vi "example_01_binary_tree.vi"(8 "error in (no error)":errorcluster) -> (0 "error out":errorcluster)   [LabVIEW 2015, in "binary_tree.lvlib"]
uses:
  binary_tree.lvlib
panel:
  in  "Delete Data":bool
  out "Data (Found)":bool
  out "Data (search)":dbl
  out "Updated?":bool
  out "Inserted?":bool
  in  "search (key)":dbl
  in  "Search Data":bool
  in  "Vizualize Data":bool
  in  "Generate Data":bool
  out "Tree [[]]":dbl[][](array[numeric])
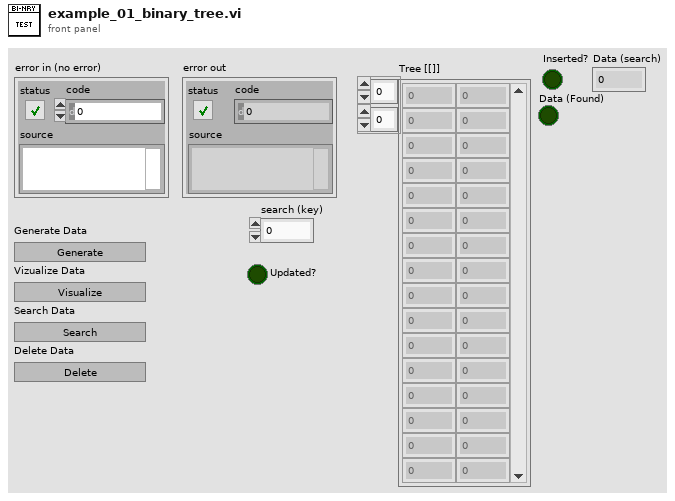
[diagram p1: front panel]
types:
  T1 = typedef "binary_tree.lvlib/node_data.ctl" = cluster{dbl}
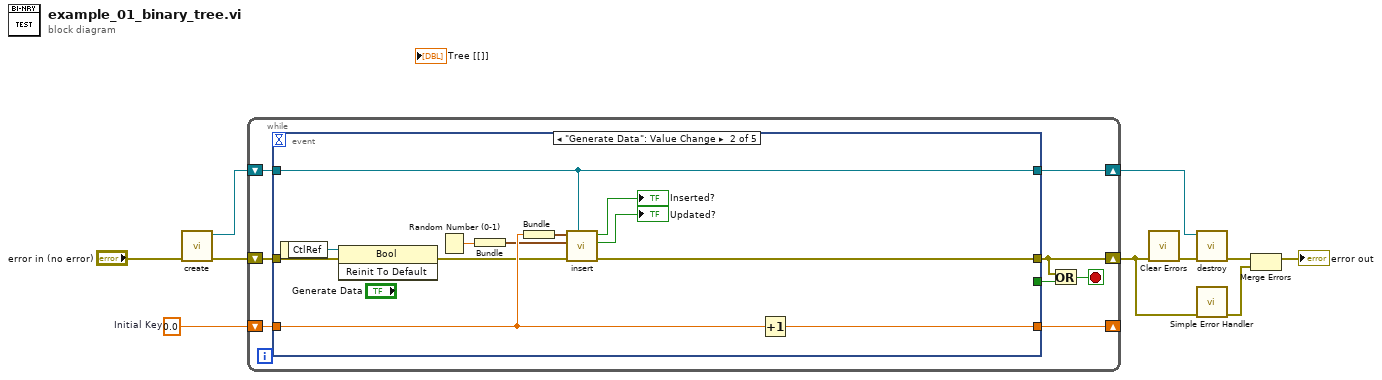
[diagram p0: block diagram]
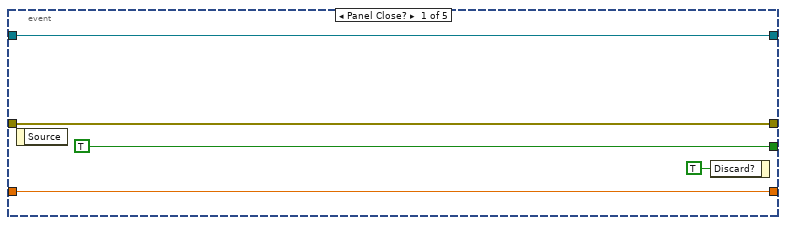
[diagram p2: hidden frame]
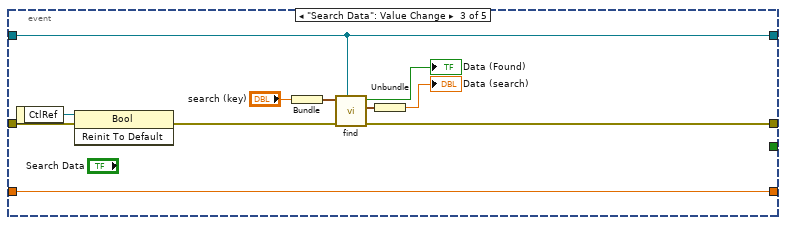
[diagram p3: hidden frame]
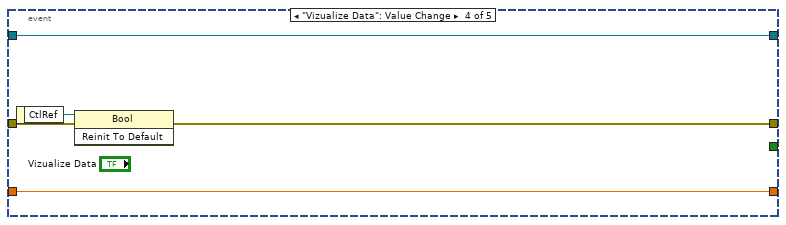
[diagram p4: hidden frame]
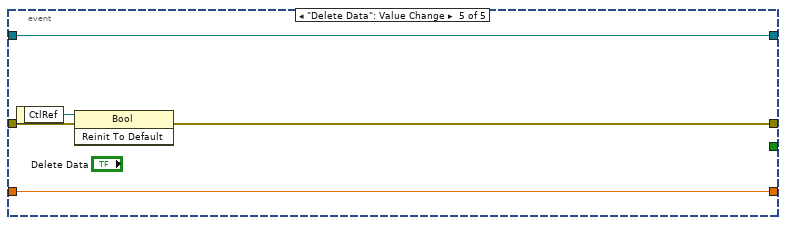
[diagram p5: hidden frame]
diagram:
  w10 = 0.0  # Initial Key
  n1 = call "create.vi"("error in (no error)"="error in (no error)") -> ("error out"=w8:errorcluster, "tree (dvr)"=w7:refnum<data-value>)  [unwired: 9 in]
  n2 = while {
    shift-right: [w15] -> w2
    shift-left: w8 -> [w18]
    shift-right: [w13] -> _
    shift-left: w10 -> [w14]
    shift-right: [w11] -> w5
    shift-left: w7 -> [w12]
    stop <- w16 stop-if-true
    n3 = event shown="[1] \"Generate Data\": Value Change" {
      selector: _ -> [_ _ _ _ _]
      dyn-events: _ -> [_ _ _ _ _]
      timeout: _ -> [_ _ _ _ _]
      tunnel: [TRUE _ _ _ _] -> w17
      tunnel: w18 -> [w21 w34 w45 w50 w55]
      tunnel: [w21 w26 w42 w47 w52] -> w15
      tunnel: w14 -> [w20 w31 w44 w49 w54]
      tunnel: [w20 w33 w44 w49 w54] -> w13
      tunnel: w12 -> [w19 w27 w41 w48 w53]
      tunnel: [w19 w27 w41 w48 w53] -> w11
      event Panel Close? {
        n4 = event-data() -> ()  [unwired: 1 in, 1 out]
        n5 = event-data("Discard?"=TRUE) -> ()  [unwired: 1 in, 1 out]
      }
      event "Generate Data": Value Change {
        n6 = event-data() -> ("CtlRef"=w35:refnum<vi>)  [unwired: 1 in]
        n7 = invoke class="Bool" method="Reinit To Default"(reference=w35, error in=w34) -> (error out=w28:errorcluster)  [unwired: 1 in, 2 out]
        n8 = Random Number (0-1)() -> (number: 0 to 1=w29:dbl)
        n9 = Bundle("number: 0 to 1"=w29) -> (w30:cluster{"number: 0 to 1":dbl})  [unwired: 1 in]
        n10 = Bundle("Initial Key"=w31) -> (w32:cluster{"Initial Key":dbl})  [unwired: 1 in]
        n11 = call "insert.vi"("tree (dvr) in"=w27, "error in (no error)"=w28, "Data"=w30, "Key"=w32) -> ("error out"=w26:errorcluster, "Updated?"=→"Updated?":bool, "Inserted?"=→"Inserted?":bool)  [unwired: 5 in]
        n12 = Increment(x=w31) -> (x+1=w33:dbl)
      }
      event "Search Data": Value Change {
        n13 = event-data() -> ("CtlRef"=w46:refnum<vi>)  [unwired: 1 in]
        n14 = invoke class="Bool" method="Reinit To Default"(reference=w46, error in=w45) -> (error out=w43:errorcluster)  [unwired: 1 in, 2 out]
        n15 = Bundle("search (key)"="search (key)") -> (w39:cluster{"search (key)":dbl})  [unwired: 1 in]
        n16 = call "find.vi"("tree (dvr) in"=w41, "error in (no error)"=w43, "Key (search)"=w39) -> ("error out"=w42:errorcluster, "Data"=w38:T1, "Found?"=→"Data (Found)":bool)  [unwired: 6 in]
        n17 = Unbundle(w38) -> (→"Data (search)":dbl)
      }
      event "Vizualize Data": Value Change {
        n18 = event-data() -> ("CtlRef"=w51:refnum<vi>)  [unwired: 1 in]
        n19 = invoke class="Bool" method="Reinit To Default"(reference=w51, error in=w50) -> (error out=w47:errorcluster)  [unwired: 1 in, 2 out]
      }
      event "Delete Data": Value Change {
        n20 = event-data() -> ("CtlRef"=w56:refnum<vi>)  [unwired: 1 in]
        n21 = invoke class="Bool" method="Reinit To Default"(reference=w56, error in=w55) -> (error out=w52:errorcluster)  [unwired: 1 in, 2 out]
      }
    }
    n22 = Or(x=w15, y=w17) -> (x .or. y?=w16:bool)
  }
  n23 = call <vilib>:"Clear Errors.vi"("error in (no error)"=w2) -> ("error out"=w6:errorcluster)  [unwired: 5 in, 1 out]
  n24 = call "destroy.vi"("error in (no error)"=w6, "tree (dvr)"=w5) -> ("error []"=w4:errorcluster[])  [unwired: 9 in]
  n25 = call <vilib>:"Simple Error Handler.vi"("error in (no error)"=w2) -> ("error out"=w1:errorcluster)  [unwired: 4 in, 4 out]
  n26 = Merge Errors(w4, w1) -> (→"error out":errorcluster)
